vi "DB Close.vi"(8 "error in":errorcluster, 11 "Database in":refnum<class "SQLite Database.lvclass">) -> (0 "error out":errorcluster, 3 "Database out":refnum<class "SQLite Database.lvclass">)   [LabVIEW 2023, in "HardwareAbstractionLayer_LVOOP.lvlib" / "SQLite Database.lvclass"]
doc: "This VI is Database Close Reference"
uses:
  SQLite Database.lvclass
  SQLite Database.lvclass/SQLite Database.ctl
  <vilib>/addons/database/NI_Database_API.lvlib
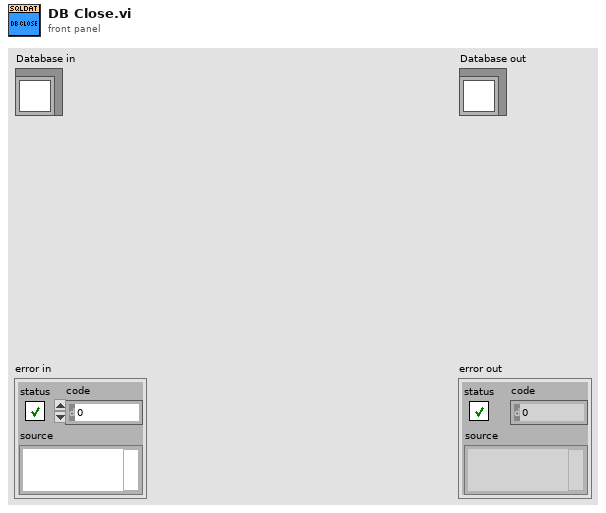
[diagram p1: front panel]
types:
  T1 = typedef "NI_Database_API.lvlib/Conn ObjectReference.ctl" = refnum<k1>
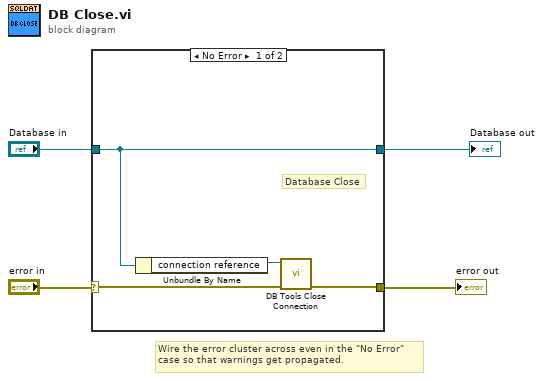
[diagram p0: block diagram]
diagram:
  # "Wire the error cluster across even in the \"No Error\"\ncase so that warnings get propagated."
  n1 = case shown="No Error" "error in" {
    selector: "error in" -> [w6 w10]
    tunnel: [w5 w10] -> w3
    tunnel: [w8 w9] -> w1
    tunnel: "Database in" -> [w8 w9]
    frame No Error {
      # "Database Close"
      n2 = Unbundle By Name(w8) -> ("connection reference"=w7:T1)
      n3 = call <vilib>:"DB Tools Close Connection.vi"("error in (no error)"=w6, "connection reference"=w7) -> ("error out"=w5:errorcluster)  [unwired: 5 in]
    }
    frame Error {
    }
  }
  "error out" <- w3
  "Database out" <- w1
